vi "Fridge_Valve_Main.vi"(8 "cluster_ref_fridge_valve":T1) -> ()   [LabVIEW 2019]
uses:
  cluster_ref_fridge_valve.ctl
  C:/Program Files/National Instruments/LabVIEW 2019/vi.lib/ULx/ULx_LV.dll
  Program Files/National Instruments/LabVIEW 2019/vi.lib/ULx/ULx_LV.dll
panel:
  out "B.V. Opening Slide":dbl(slide) scale=0.0..100.0
  out "R.V. Opening Slide":dbl(slide) scale=0.0..100.0
  in  "Automated\nRun-Valve\nControl":bool
  in  "R.V. \nMotor\nPower":bool=TRUE
  in  "Set RV Opening":dbl caption="Set Opening"
  out "R.V. Motor Status":bool
  in  "R.V. VISA":refnum<visa-resource-name>="COM9"
  out "He Level":waveform(dbl)[](graph)
  out "He Level":dbl(slide) scale=0.0..100.0
  out "Level Probe Status":bool
  in  "AMI1700 VISA":refnum<visa-resource-name>="COM11"
  in  "Set BV Opening":dbl caption="Set Opening"
  out "B.V. Init Step":i32
  out "R.V. Init Step":i32
  out "Run Valve Steps":i32 caption="Motor Step"
  out "Run Valve ADC":dbl caption="ADC"
  out "Bypass Valve ADC":dbl caption="ADC"
  out "Bypass Valve Step":i32 caption="Motor Step"
  out "Bypass Valve Opening":waveform(dbl)[](graph)
  out "Run Valve Opening":waveform(dbl)[](graph)
  out "ADC Status":bool=TRUE
  out "Last Updated":timestamp format="%<%Y-%m-%d %H:%M:%S>T"
  in  "B.V. VISA":refnum<visa-resource-name>="COM22"
  in  "B.V.\nMotor\nPower":bool=TRUE
  in  "Stop":bool
  in  "Pause":bool=TRUE
  out "B.V. Motor Status":bool
  in  "Enable Advanced Controls":bool
  # "Fridge Valve Panel"
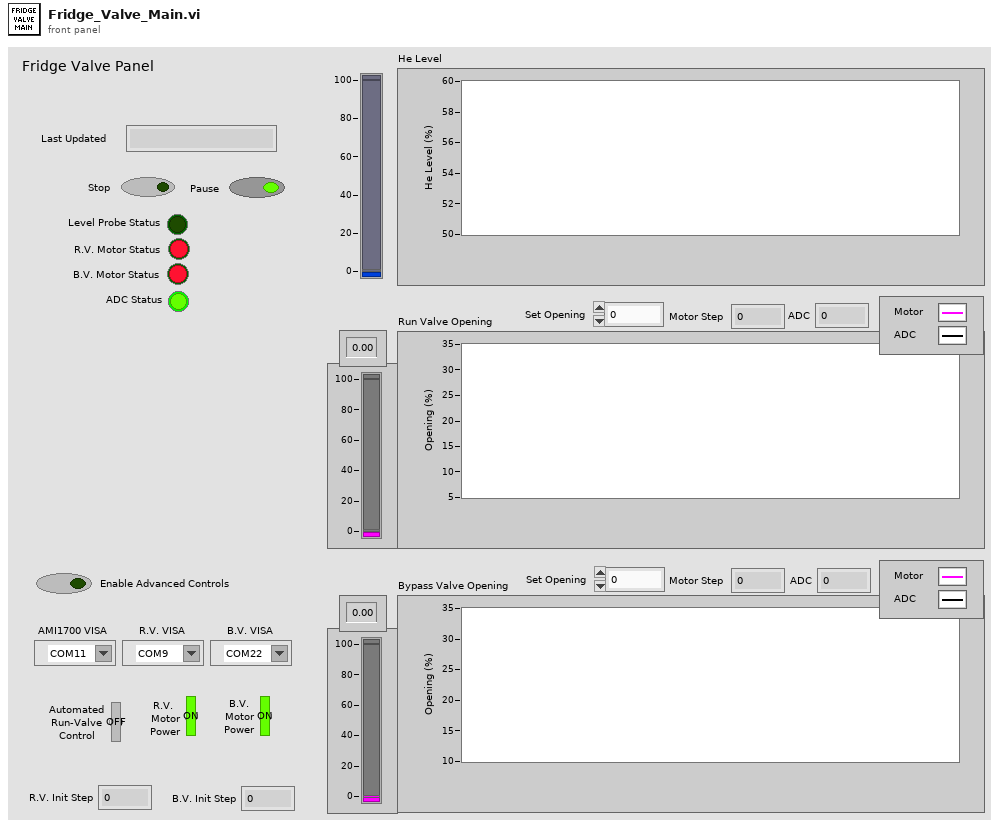
[diagram p1: front panel]
types:
  T1 = typedef "cluster_ref_fridge_valve.ctl" = cluster{"Status":refnum<vi>, "RVO":refnum<vi>, "BVO":refnum<vi>, "He Level":refnum<vi>}
  T2 = enum8{"Enabled", "Disabled", "Disabled and Grayed Out"}
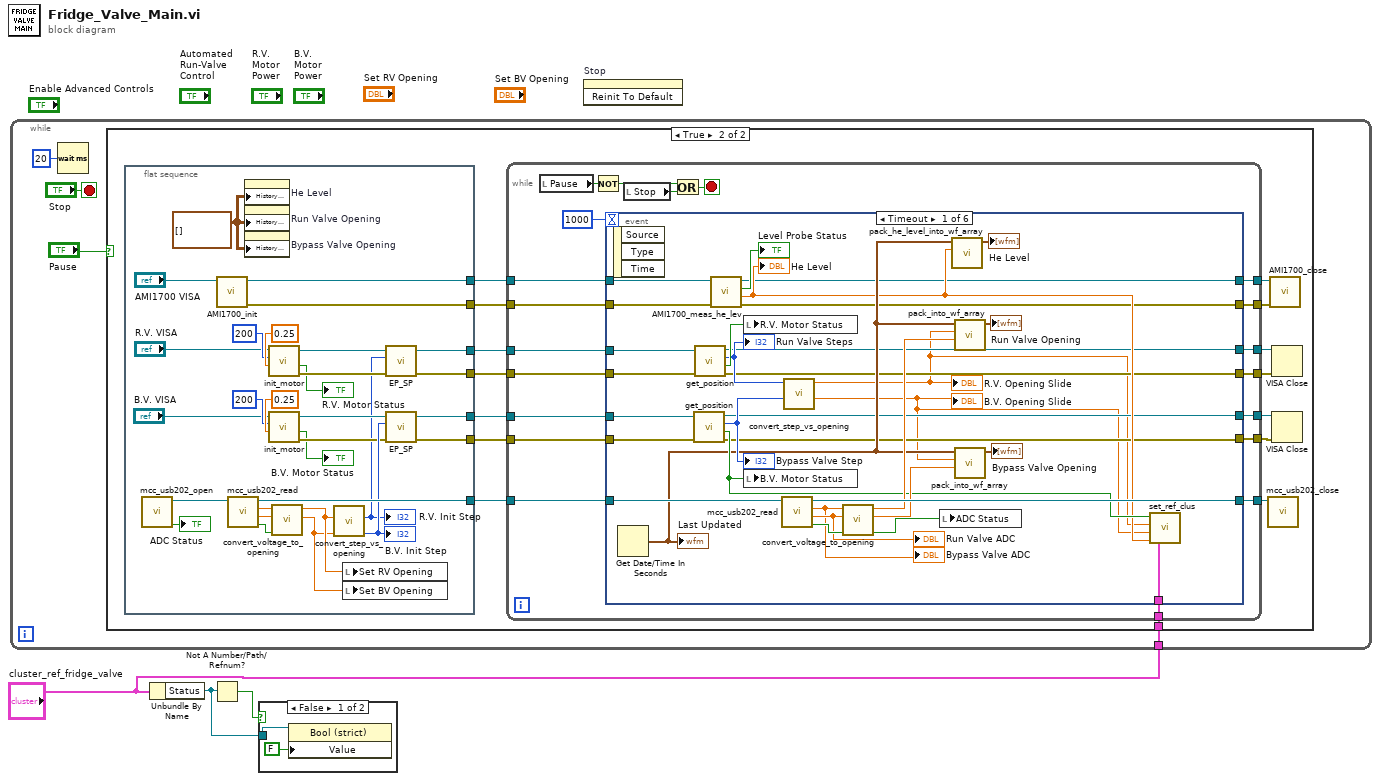
[diagram p0: block diagram]
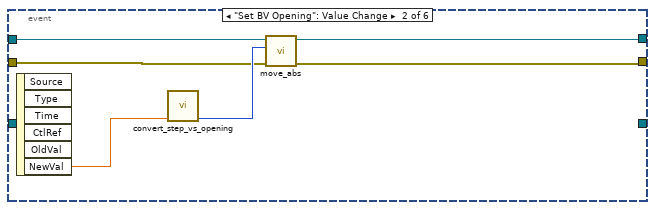
[diagram p4: hidden frame]
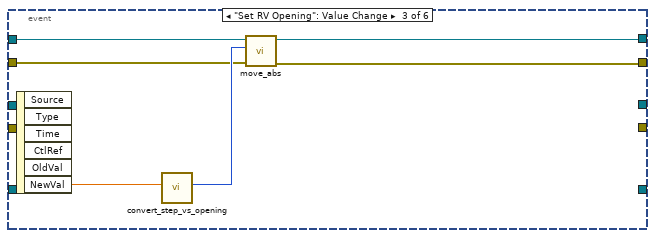
[diagram p5: hidden frame]
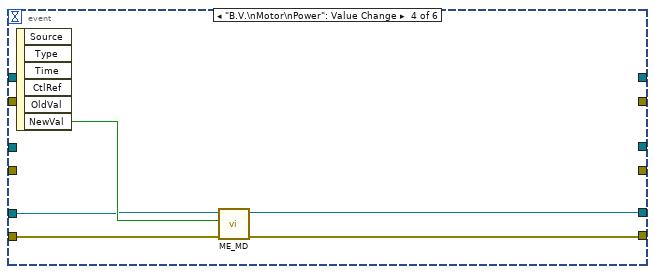
[diagram p6: hidden frame]
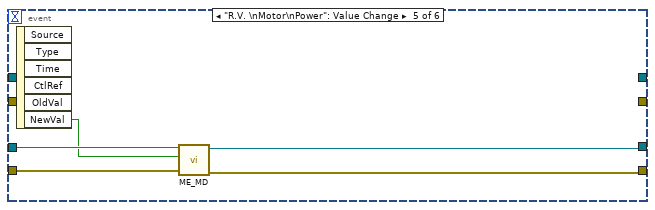
[diagram p7: hidden frame]
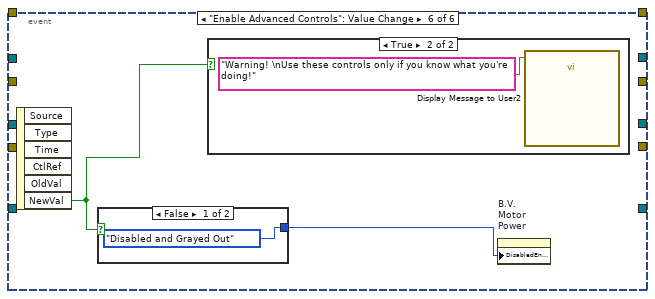
[diagram p8: hidden frame]
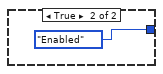
[diagram p9: hidden frame]
diagram:
  n1 = while {
    tunnel: "cluster_ref_fridge_valve" -> [w4]
    stop <- "Stop" stop-if-true
    n2 = Wait (ms)(milliseconds to wait=u32 20) -> ()  [unwired: 1 out]
    n3 = case shown="True" "Pause" {
      tunnel: w4 -> [_ w18]
      frame False {
      }
      frame True {
        n4 = flat-sequence {
          tunnel: [w45] -> w22
          tunnel: [w50] -> w21
          tunnel: [w44] -> w19
          tunnel: [w36] -> w17
          tunnel: [w35] -> w16
          tunnel: [w28] -> w15
          tunnel: [w27] -> w14
          frame #0 {
            w25 = waveform(dbl)[][] [] ("History Data")
            n5 = call "mcc_usb202_open.vi"() -> ("status"=→"ADC Status":bool, "task out"=w51:refnum<k24>)  [unwired: 9 in, 1 out]
            n6 = call "AMI1700_init.vi"("VISA in"="AMI1700 VISA") -> ("error out"=w36:errorcluster, "VISA out"=w35:refnum<visa-resource-name>)  [unwired: 9 in]
            n7 = call "mcc_usb202_read.vi"("task in"=w51) -> ("status"=w47:bool, "V1"=w48:dbl, "V0"=w49:dbl, "task out"=w50:refnum<k24>)  [unwired: 6 in, 1 out]
            n8 = property on="He Level" class="WFChart (strict)"("History Data"=w25) -> ()  [unwired: 2 in, 2 out]
            n9 = property on="Run Valve Opening" class="WFChart (strict)"("History Data"=w25) -> ()  [unwired: 2 in, 2 out]
            n10 = property on="Bypass Valve Opening" class="WFChart (strict)"("History Data"=w25) -> ()  [unwired: 2 in, 2 out]
            n11 = call "init_motor.vi"("velocity"=0.25, "steps_per_rev"=200, "VISA in"="R.V. VISA") -> ("error out"=w31:errorcluster, "status"=→"R.V. Motor Status":bool, "VISA out"=w32:refnum<visa-resource-name>)  [unwired: 6 in]
            n12 = call "init_motor.vi"("velocity"=0.25, "steps_per_rev"=200, "VISA in"="B.V. VISA") -> ("error out"=w39:errorcluster, "status"=→"B.V. Motor Status":bool, "VISA out"=w40:refnum<visa-resource-name>)  [unwired: 6 in]
            n13 = call "convert_voltage_to_opening.vi"("status_in"=w47, "bypass_valve_voltage"=w48, "run_valve_voltage"=w49) -> ("bypass_valve_opening"=w23:dbl, "run_valve_opening"=w24:dbl)  [unwired: 6 in, 1 out]
            n14 = call "convert_step_vs_opening.vi"("bypass_valve_opening_in"=w23, "run_valve_opening_in"=w24) -> ("bypass_valve_step_out"=w46:i32, "run_valve_step_out"=w26:i32)  [unwired: 6 in, 2 out]
            "R.V. Init Step" <- w26
            "B.V. Init Step" <- w46
            n15 = local write "Set RV Opening"(w24) -> ()
            n16 = local write "Set BV Opening"(w23) -> ()
            n17 = call "EP_SP.vi"("error in"=w31, "new_position"=w26, "VISA in"=w32) -> ("error out"=w28:errorcluster, "VISA out"=w27:refnum<visa-resource-name>)  [unwired: 7 in]
            n18 = call "EP_SP.vi"("error in"=w39, "new_position"=w46, "VISA in"=w40) -> ("error out"=w45:errorcluster, "VISA out"=w44:refnum<visa-resource-name>)  [unwired: 7 in]
          }
        }
        n19 = while {
          tunnel: w22 -> [w70]
          tunnel: w19 -> [w64]
          tunnel: w21 -> [w68]
          tunnel: [w67] -> w20
          tunnel: w18 -> [w63]
          tunnel: w17 -> [w62]
          tunnel: w16 -> [w61]
          tunnel: w15 -> [w60]
          tunnel: w14 -> [w59]
          tunnel: [w58] -> w13
          tunnel: [w57] -> w12
          tunnel: [w56] -> w11
          tunnel: [w55] -> w10
          tunnel: [w54] -> w9
          tunnel: [w53] -> w8
          stop <- w71 stop-if-true
          n20 = local read "Pause"() -> (w72:bool)
          n21 = Not(x=w72) -> (.not. x?=w66:bool)
          n22 = event shown="[0] Timeout" {
            selector: _ -> [_ _ _ _ _ _]
            dyn-events: _ -> [_ _ _ _ _ _]
            timeout: 1000 -> [_ _ _ _ _ _]
            tunnel: w64 -> [w95 w110 _ w120 _ _]
            tunnel: w70 -> [w94 w108 _ w121 _ _]
            tunnel: w68 -> [w105 _ _ _ _ _]
            tunnel: [w103 _ _ _ _ _] -> w67
            tunnel: w63 -> [w92 _ _ _ _ _]
            tunnel: w62 -> [w89 _ _ _ _ _]
            tunnel: w61 -> [w88 _ _ _ _ _]
            tunnel: w60 -> [w84 _ w114 _ w126 _]
            tunnel: w59 -> [w83 _ w115 _ w127 _]
            tunnel: [w80 _ _ _ _ _] -> w58
            tunnel: [w79 _ _ _ _ _] -> w57
            tunnel: [w78 w107 _ w119 _ _] -> w56
            tunnel: [w77 w106 _ w118 _ _] -> w55
            tunnel: [w76 _ w113 _ w124 _] -> w54
            tunnel: [w75 _ w112 _ w125 _] -> w53
            event Timeout {
              n23 = event-data() -> ()  [unwired: 1 in, 3 out]
              n24 = Get Date/Time In Seconds() -> (seconds since 1Jan1904=w86:timestamp)
              "Last Updated" <- w86
              n25 = call "get_position.vi"("error in (no error)"=w94, "VISA resource name"=w95) -> ("error out"=w77:errorcluster, "status"=w91:bool, "Position"=w93:i32, "VISA resource name 2"=w78:refnum<visa-resource-name>)  [unwired: 6 in]
              "Bypass Valve Step" <- w93
              n26 = call "get_position.vi"("error in (no error)"=w84, "VISA resource name"=w83) -> ("error out"=w75:errorcluster, "status"=w82:bool, "Position"=w81:i32, "VISA resource name 2"=w76:refnum<visa-resource-name>)  [unwired: 6 in]
              "Run Valve Steps" <- w81
              n27 = call "AMI1700_meas_he_lev.vi"("error in"=w89, "VISA in"=w88) -> ("error out"=w79:errorcluster, "level"=w85:dbl, "status"=→"Level Probe Status":bool, "VISA out"=w80:refnum<visa-resource-name>)  [unwired: 6 in]
              "He Level" <- w85
              n28 = local write "R.V. Motor Status"(w82) -> ()
              n29 = local write "B.V. Motor Status"(w91) -> ()
              n30 = call "mcc_usb202_read.vi"("task in"=w105) -> ("status"=w104:bool, "V1"=w98:dbl, "V0"=w97:dbl, "task out"=w103:refnum<k24>)  [unwired: 6 in, 1 out]
              "Bypass Valve ADC" <- w98
              "Run Valve ADC" <- w97
              n31 = call "convert_step_vs_opening.vi"("bypass_valve_step_in"=w93, "run_valve_step_in"=w81) -> ("bypass_valve_opening_out"=w73:dbl, "run_valve_opening_out"=w74:dbl)  [unwired: 6 in, 2 out]
              "R.V. Opening Slide" <- w74
              "B.V. Opening Slide" <- w73
              n32 = call "convert_voltage_to_opening.vi"("status_in"=w104, "bypass_valve_voltage"=w98, "run_valve_voltage"=w97) -> ("status_out"=w96:bool, "bypass_valve_opening"=w101:dbl, "run_valve_opening"=w99:dbl)  [unwired: 6 in]
              n33 = local write "ADC Status"(w96) -> ()
              n34 = call "pack_he_level_into_wf_array.vi"("he_level"=w85, "time"=w86) -> ("waveform_array"=→"He Level":waveform(dbl)[])  [unwired: 9 in]
              n35 = call "pack_into_wf_array.vi"("value_adc"=w99, "value_motor"=w74, "time"=w86) -> ("waveform_array"=→"Run Valve Opening":waveform(dbl)[])  [unwired: 8 in]
              n36 = call "pack_into_wf_array.vi"("value_adc"=w101, "value_motor"=w73, "time"=w86) -> ("waveform_array"=→"Bypass Valve Opening":waveform(dbl)[])  [unwired: 8 in]
              n37 = call "set_ref_clus.vi"("cluster_ref"=w92, "he_level"=w85, "bypass_valve_opening"=w73, "run_valve_opening"=w74, "status"=w91) -> ()  [unwired: 7 in]
            }
            event "Set BV Opening": Value Change {
              n38 = event-data() -> ("NewVal"=w111:dbl)  [unwired: 1 in, 5 out]
              n39 = call "convert_step_vs_opening.vi"("bypass_valve_opening_in"=w111) -> ("bypass_valve_step_out"=w109:i32)  [unwired: 7 in, 3 out]
              n40 = call "move_abs.vi"("error in"=w108, "Position Aboslute"=w109, "VISA in"=w110) -> ("error out"=w106:errorcluster, "VISA out"=w107:refnum<visa-resource-name>)  [unwired: 7 in]
            }
            event "Set RV Opening": Value Change {
              n41 = event-data() -> ("NewVal"=w117:dbl)  [unwired: 1 in, 5 out]
              n42 = call "convert_step_vs_opening.vi"("run_valve_opening_in"=w117) -> ("run_valve_step_out"=w116:i32)  [unwired: 7 in, 3 out]
              n43 = call "move_abs.vi"("error in"=w114, "Position Aboslute"=w116, "VISA in"=w115) -> ("error out"=w112:errorcluster, "VISA out"=w113:refnum<visa-resource-name>)  [unwired: 7 in]
            }
            event "B.V.\nMotor\nPower": Value Change {
              n44 = event-data() -> ("NewVal"=w122:bool)  [unwired: 1 in, 5 out]
              n45 = call "ME_MD.vi"("error in"=w121, "enable_or_disable"=w122, "VISA in"=w120) -> ("error out"=w118:errorcluster, "VISA out"=w119:refnum<visa-resource-name>)  [unwired: 6 in, 1 out]
            }
            event "R.V. \nMotor\nPower": Value Change {
              n46 = event-data() -> ("NewVal"=w123:bool)  [unwired: 1 in, 5 out]
              n47 = call "ME_MD.vi"("error in"=w126, "enable_or_disable"=w123, "VISA in"=w127) -> ("error out"=w125:errorcluster, "VISA out"=w124:refnum<visa-resource-name>)  [unwired: 6 in, 1 out]
            }
            event "Enable Advanced Controls": Value Change {
              n48 = event-data() -> ("NewVal"=w129:bool)  [unwired: 1 in, 5 out]
              n49 = case shown="False" w129 {
                tunnel: [T2."Disabled and Grayed Out" ("Disabled") T2."Enabled" ("Disabled")] -> w128
                frame False {
                }
                frame True {
                }
              }
              n50 = case shown="True" w129 {
                frame False {
                }
                frame True {
                  n51 = call "Display Message to User2"("Message"="Warning! \nUse these controls only if you know what you're doing!") -> ()  [unwired: 9 in, 2 out]
                }
              }
              n52 = property on="B.V.\nMotor\nPower" class="Bool (strict)"("DisabledEnum"=w128) -> ()  [unwired: 2 in, 2 out]
            }
          }
          n53 = local read "Stop"() -> (w65:bool)
          n54 = Or(x=w66, y=w65) -> (x .or. y?=w71:bool)
        }
        n55 = call "mcc_usb202_close.vi"("task in"=w20) -> ()  [unwired: 9 in, 2 out]
        n56 = call "AMI1700_close.vi"("error in"=w12, "VISA in"=w13) -> ()  [unwired: 9 in, 1 out]
        n57 = VISA Close(VISA resource name=w9, error in (no error)=w8) -> ()  [unwired: 1 out]
        n58 = VISA Close(VISA resource name=w11, error in (no error)=w10) -> ()  [unwired: 1 out]
      }
    }
  }
  n59 = Unbundle By Name("cluster_ref_fridge_valve") -> ("Status"=w3:refnum<vi>)
  n60 = Not A Number/Path/Refnum?(number/path/refnum=w3) -> (NaN/Path/Refnum?=w2:bool)
  n61 = case shown="False" w2 {
    tunnel: w3 -> [w134 _]
    frame False {
      n62 = property class="Bool (strict)"(reference=w134, "Value"=FALSE) -> ()  [unwired: 1 in, 2 out]
    }
    frame True {
    }
  }
  n63 = invoke on="Stop" class="Bool (strict)" method="Reinit To Default"() -> ()  [unwired: 3 in, 3 out]
